vi "CalculateLifetime.vi"(6 "Pos Array":i32[][](array[numeric]), 7 "starting y-point":i32) -> (1 "Decay":u32[][](array[numeric]))   [LabVIEW 2009]
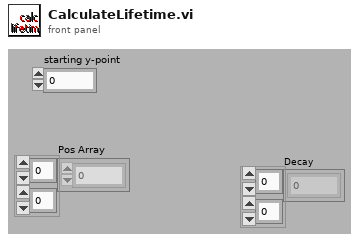
[diagram p1: front panel]
types:
  T1 = enum16{"Display", "change", "Get", "Set", "Set Ken"}
  T2 = typedef "FIFOSettings_BH.ctt" = cluster{"Measurement":cluster{"Binning (ms)":sgl, "External Trigger Condition":u16, "Stop Condition:":u16, "Stop Count":dbl, "Buffer Size (Photons)":u16, "No of Channels":u16, "Ext Latch Delay":i16}, "ADC":cluster{"Module":u16, "ADC Resolution":i32, "Dither Range":i16, "Count Increment":i16, "Macro Time Clock":i16}, "SYNC":cluster{"SYNC ZC Level (mV)":sgl, "SYNC Freq Divider":i16, "SYNC Holdoff (ns)":sgl, "SYNC Threshold (mV)":sgl}, "TAC":cluster{"TAC Range (ns)":sgl, "TAC Gain":i16, "TAC Offset (%)":sgl, "TAC Limit Low (%)":sgl, "TAC Limit High (%)":sgl}, "CFD":cluster{"CFD Limit Low (mV)":sgl, "CFD Limit High (mV)":sgl, "CFD ZC Level (mV)":sgl, "CFD Holdoff (ns)":sgl}}
  T3 = typedef "ImageSettings.ctt" = cluster{"Start Position (µm)":cluster{"x":dbl, "y":dbl, "z":dbl}, "End Position (µm)":cluster{"x":dbl, "y":dbl, "z":dbl}, "Image Resolution (nm/pixel)":cluster{"x":dbl, "y":dbl, "z":dbl}, "Image Size (µm)":cluster{"x":dbl, "y":dbl, "z":dbl}, "Image Size (pixel)":cluster{"x":u32, "y":u32, "z":u32}, "Time Resolution\n(ms/pixel)":dbl, "1st Axis":u16, "2nd Axis":u16, "Retrace":bool, "Estimated Time":string}
  T4 = typedef "Settings.ctl" = cluster{"threshold":cluster{"max":u32, "min":u32}, "RGB or false color":bool, "16bit":bool, "log/lin axis":u16, "spotsize button":bool, "Pixelsize":u16, "autoscale x":bool, "autoscale y":bool, "correlation":bool, "ADC-Resolution":i32, "F2-lifetime":cluster{"display tau":bool, "display F2":bool, "Palette Number lifetime":enum32{"Gray", "Binary", "Gradient", "Rainbow", "Temperature"}, "Palette Number F2":enum32{"Gray", "Binary", "Gradient", "Rainbow", "Temperature"}, "max tau-Value":dbl, "min tau-Value":dbl, "max F2-Value":dbl, "min F2-Value":dbl}, "TAC-Window 1":u16, "TAC-Window 2":u16, "false color palette":cluster{"1":u32, "2":u32, "3":u32, "4":u32, "5":u32, "6":u32, "7":u32, "8":u32, "8 2":u32, "8 3":u32, "8 4":u32, "8 5":u32}, "rebinning":dbl}
  T5 = cluster{"router":u8[], "macro times":dbl[], "micro times":u16[], "invalid":dbl[], "gap":dbl[]}
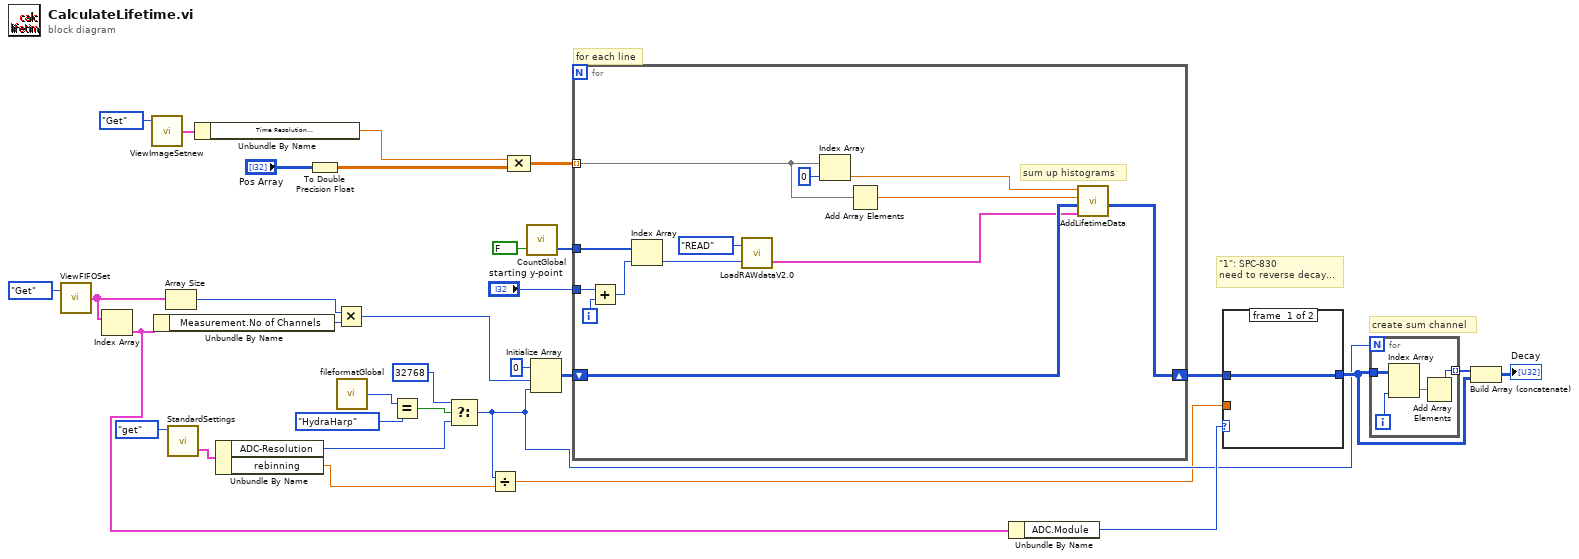
[diagram p0: block diagram]
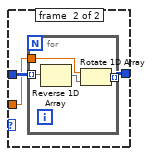
[diagram p2: hidden frame]
diagram:
  # "\"1\": SPC-830\nneed to reverse decay..."
  # "create sum channel"
  # "for each line"
  n1 = call "ViewFIFOSet.vi"("Enum"=T1."Get") -> ("FIFO Settings (Array)"=w18:T2[])  [unwired: 1 in]
  n2 = Index Array(array=w18) -> (element=w7:T2)  [unwired: 1 in]
  n3 = call "ViewImageSetnew.vi"("action"=T1."Get" ("Enum")) -> ("Image Settings"=w25:T3)  [unwired: 2 in]
  n4 = Unbundle By Name(w7) -> ("Measurement.No of Channels"=w17:u16)
  n5 = Array Size(array=w18) -> (size(s)=w16:i32)
  n6 = call "StandardSettings.vi"("Enum"=enum16{"Load", "get", "Save", "set"}."get") -> ("StandardSettings"=w20:T4)  [unwired: 4 in]
  n7 = Unbundle By Name(w25) -> ("Time Resolution\n(ms/pixel)"=w23:dbl)
  n8 = Unbundle By Name(w20) -> ("ADC-Resolution"=w9:i32, "rebinning"=w2:dbl)
  n9 = To Double Precision Float(number="Pos Array") -> (double precision float=w22:dbl[][])
  n10 = Multiply(x=w16, y=w17) -> (x*y=w15:i32)
  n11 = call "fileformatGlobal.vi"() -> ("fileformat out"=w12:enum16{"Herty", "Ken", "SPC130", "HydraHarp"})  [unwired: 2 in]
  n12 = Equal?(x=w12, y=enum16{"Herty", "Ken", "SPC130", "HydraHarp"}."HydraHarp") -> (x = y?=w10:bool)
  n13 = Select(t=32768, s=w10, f=w9) -> (s? t:f=w3:i32)
  n14 = Divide(x=w3, y=w2) -> (x/y=w1:dbl)
  n15 = Compound Arithmetic op=MULTIPLY(w23, w22) -> (w14:dbl[][])
  n16 = call "CountGlobal.vi"("changed?"=FALSE) -> ("count out"=w31:i32[])  [unwired: 2 in]
  n17 = Initialize Array(u32 0 ("element"), w15, w3) -> (w28:u32[][])
  n18 = for {
    tunnel: "starting y-point" -> [w44]
    tunnel: w14 -> [w42] mode=indexing
    tunnel: w31 -> [w41]
    shift-right: [w34] -> w6
    shift-left: w28 -> [w35]
    i -> [w43]
    # "sum up histograms"
    n19 = Add(x=w44, y=w43) -> (x+y=w39:i32)
    n20 = Index Array(array=w41, index=w39) -> (element=w40:i32)
    n21 = call "LoadRAWdataV2.0.vi"("pos offset (0)"=w40, "action"=enum16{"OPEN", "READ", "CLOSE"}."READ" ("Enum")) -> ("RAW data"=w33:T5)  [unwired: 1 out]
    n22 = Index Array(array=w42, index=0) -> (element=w37:dbl)
    n23 = Add Array Elements(numeric array=w42) -> (sum=w36:dbl)
    n24 = call "AddLifetimeData.vi"("lower time (ms)"=w37, "upper time (ms)"=w36, "Decay"=w35, "RAW data"=w33) -> ("Decay out"=w34:u32[][])  [unwired: 5 in]
  }
  n25 = Unbundle By Name(w7) -> ("ADC.Module"=w4:u16)
  n26 = case shown="1" w4 {
    tunnel: w6 -> [w46 w49]
    tunnel: [w46 w47] -> w5
    tunnel: w1 -> [_ w48]
    frame #0 {
    }
    frame #1 {
      n27 = for {
        tunnel: w49 -> [w53] mode=indexing
        tunnel: w48 -> [w50]
        tunnel: [w51] -> w47 mode=indexing
        n28 = Reverse 1D Array(array=w53) -> (reversed array=w52:u32[])
        n29 = Rotate 1D Array(1:w52, 2:w50) -> (0:w51:u32[])
      }
    }
  }
  n30 = for {
    N: w3 -> [_]
    tunnel: w5 -> [w57]
    tunnel: [w54] -> w19 mode=indexing
    i -> [w56]
    n31 = Index Array(array=w57, index (col)=w56) -> (element=w55:u32[])  [unwired: 1 in]
    n32 = Add Array Elements(numeric array=w55) -> (sum=w54:u32)
  }
  n33 = Build Array (concatenate)(w19, w5) -> (→"Decay":u32[][])
